vi "ReadOperationMode(test).vi"(8 "error in":errorcluster, 10 "ON/OFF":bool, 11 "VISA resource name in":refnum<visa-resource-name>) -> (0 "error out":errorcluster, 2 "Operation Mode Status":T1, 3 "VISA resource name out":refnum<visa-resource-name>, 5 "StartOM":string)   [LabVIEW 2014]
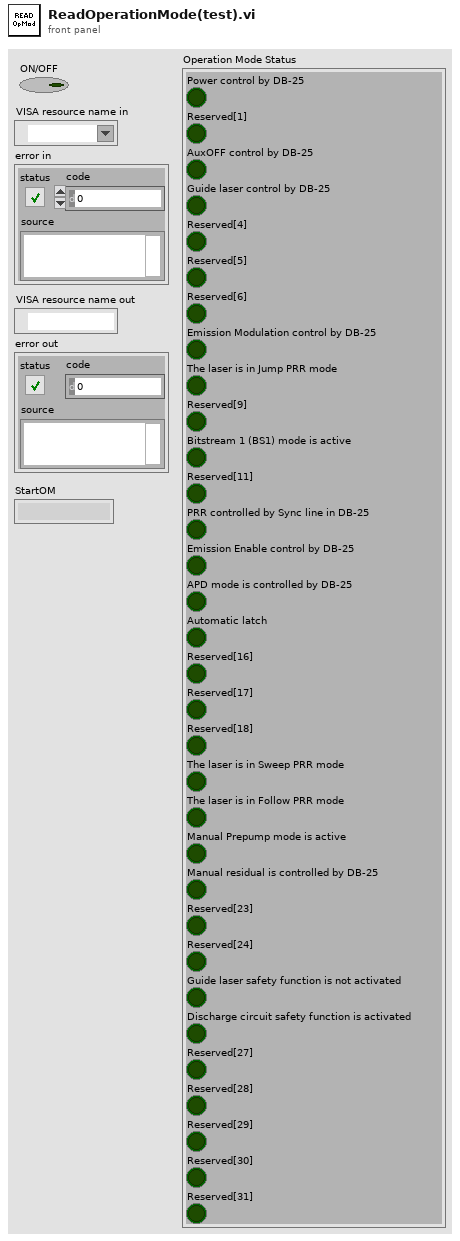
[diagram p1: front panel]
types:
  T1 = cluster{"Power control by DB-25":bool, "Reserved[1]":bool, "AuxOFF control by DB-25":bool, "Guide laser control by DB-25":bool, "Reserved[4]":bool, "Reserved[5]":bool, "Reserved[6]":bool, "Emission Modulation control by DB-25":bool, "The laser is in Jump PRR mode":bool, "Reserved[9]":bool, "Bitstream 1 (BS1) mode is active":bool, "Reserved[11]":bool, "PRR controlled by Sync line in DB-25":bool, "Emission Enable control by DB-25":bool, "APD mode is controlled by DB-25":bool, "Automatic latch":bool, "Reserved[16]":bool, "Reserved[17]":bool, "Reserved[18]":bool, "The laser is in Sweep PRR mode":bool, "The laser is in Follow PRR mode":bool, "Manual Prepump mode is active":bool, "Manual residual is controlled by DB-25":bool, "Reserved[23]":bool, "Reserved[24]":bool, "Guide laser safety function is not activated":bool, "Discharge circuit safety function is activated":bool, "Reserved[27]":bool, "Reserved[28]":bool, "Reserved[29]":bool, "Reserved[30]":bool, "Reserved[31]":bool}
  T2 = cluster{"Boolean array[0]":bool, "Boolean array[1]":bool, "Boolean array[2]":bool, "Boolean array[3]":bool, "Boolean array[4]":bool, "Boolean array[5]":bool, "Boolean array[6]":bool, "Boolean array[7]":bool, "Boolean array[8]":bool, "Boolean array[9]":bool, "Boolean array[10]":bool, "Boolean array[11]":bool, "Boolean array[12]":bool, "Boolean array[13]":bool, "Boolean array[14]":bool, "Boolean array[15]":bool, "Boolean array[16]":bool, "Boolean array[17]":bool, "Boolean array[18]":bool, "Boolean array[19]":bool, "Boolean array[20]":bool, "Boolean array[21]":bool, "Boolean array[22]":bool, "Boolean array[23]":bool, "Boolean array[24]":bool, "Boolean array[25]":bool, "Boolean array[26]":bool, "Boolean array[27]":bool, "Boolean array[28]":bool, "Boolean array[29]":bool, "Boolean array[30]":bool, "Boolean array[31]":bool}
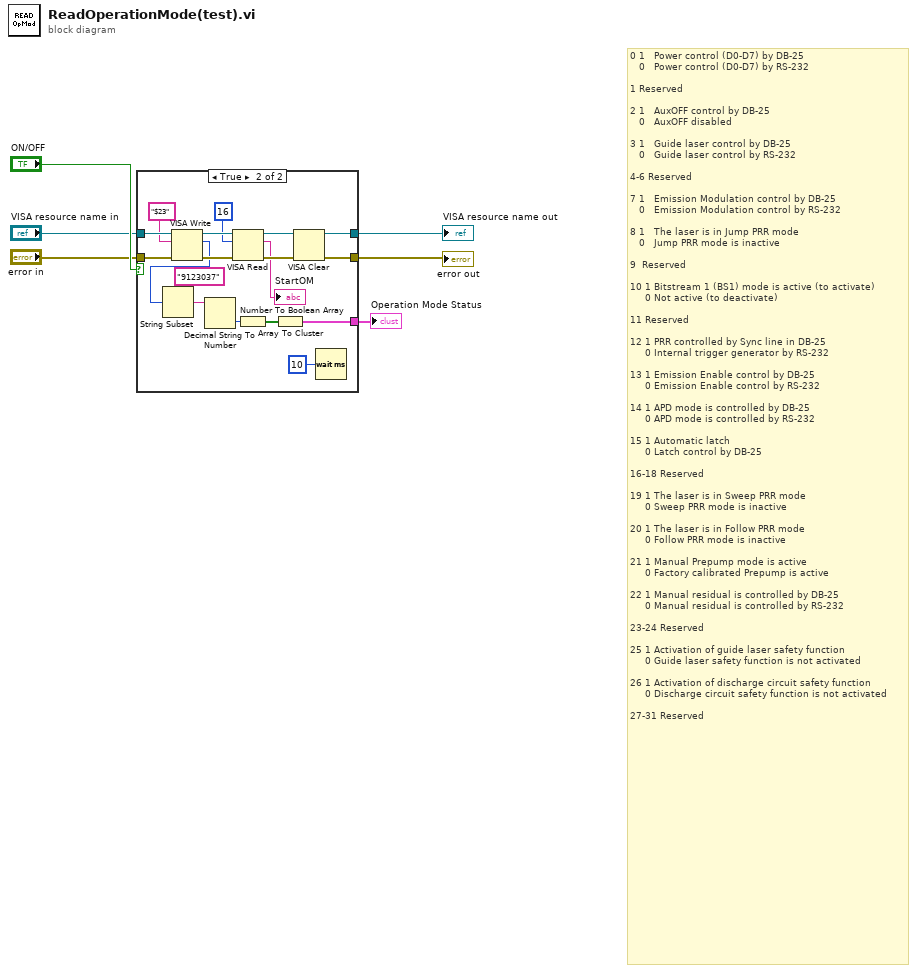
[diagram p0: block diagram]
diagram:
  # "0 1   Power control (D0-D7) by DB-25\n   0   Power control (D0-D7) by RS-232\n\n1 Reserved\n\n2 1   AuxOFF control by DB-25\n   0   AuxOFF disabled\n\n3 1   Guide laser control by DB-25\n   0   Guide laser control by RS-232\n\n4-6 Reserved\n\n7 1   Emission Modulation control by DB-25\n   0   Emission Modulation control by RS-232\n\n8 1   The laser is in Jump PRR mode\n   0   Jump PRR mode is inactive\n\n9  Reserved\n\n10 1 Bitstream 1 (BS1) mode is active (to activate)\n     0 Not active (to deactivate)\n\n11 Reserved\n\n12 1 PRR controlled by Sync line in DB-25\n     0 Internal trigger generator by RS-232\n\n13 1 Emission Enable control by DB-25\n     0 Emission Enable control by RS-232\n\n14 1 APD mode is controlled by DB-25\n     0 APD mode is controlled by RS-232\n\n15 1 Automatic latch\n     0 Latch control by DB-25\n\n16-18 Reserved\n\n19 1 The laser is in Sweep PRR mode\n     0 Sweep PRR mode is inactive\n\n20 1 The laser is in Follow PRR mode\n     0 Follow PRR mode is inactive\n\n21 1 Manual Prepump mode is active\n     0 Factory calibrated Prepump is active\n\n22 1 Manual residual is controlled by DB-25\n     0 Manual residual is controlled by RS-232\n\n23-24 Reserved\n\n25 1 Activation of guide laser safety function\n     0 Guide laser safety function is not activated\n\n26 1 Activation of discharge circuit safety function\n     0 Discharge circuit safety function is not activated\n\n27-31 Reserved"
  n1 = case shown="True" "ON/OFF" {
    tunnel: "VISA resource name in" -> [w8 w24]
    tunnel: "error in" -> [w7 w23]
    tunnel: [w8 w19] -> w3
    tunnel: [w7 w18] -> w2
    tunnel: [_ w10] -> w1
    frame False {
    }
    frame True {
      n2 = VISA Write(VISA resource name=w24, write buffer="$23", error in (no error)=w23) -> (VISA resource name out=w25:refnum<visa-resource-name>, return count=w11:u32, error out=w26:errorcluster)
      n3 = String Subset(string="9123037", offset (0)=w11) -> (substring=w13:string)  [unwired: 1 in]
      n4 = Decimal String To Number(string=w13) -> (number=w14:i32)  [unwired: 2 in, 1 out]
      n5 = VISA Read(VISA resource name=w25, byte count=u32 16, error in (no error)=w26) -> (VISA resource name out=w21:refnum<visa-resource-name>, read buffer=→"StartOM":string, error out=w20:errorcluster)  [unwired: 1 out]
      n6 = Number To Boolean Array(number=w14) -> (Boolean array=w15:bool[])
      n7 = Array To Cluster(array=w15) -> (cluster=w10:T2)
      n8 = VISA Clear(VISA resource name=w21, error in (no error)=w20) -> (VISA resource name out=w19:refnum<visa-resource-name>, error out=w18:errorcluster)
      n9 = Wait (ms)(milliseconds to wait=u32 10) -> ()  [unwired: 1 out]
    }
  }
  "VISA resource name out" <- w3
  "error out" <- w2
  "Operation Mode Status" <- w1
